vi "Constants.vi"() -> ()   [LabVIEW 2020, in "Ballard MIL-STD-1553 Shared.lvlib"]
doc: "Use this Global VI to access the GUIDs assigned to the page resources of the Custom Device."
uses:
  Ballard MIL-STD-1553 Shared.lvlib
panel:
  in  "Tab Control":enum32{"GUIDs", "Constants", "Properties"}(tab)=enum."Constants"
  in  "RTM Wrapper":string="5FF42902-C783-4304-B588-1D2F1CA49C45"
  in  "Compiled.Settings":string="Compiled.Settings"
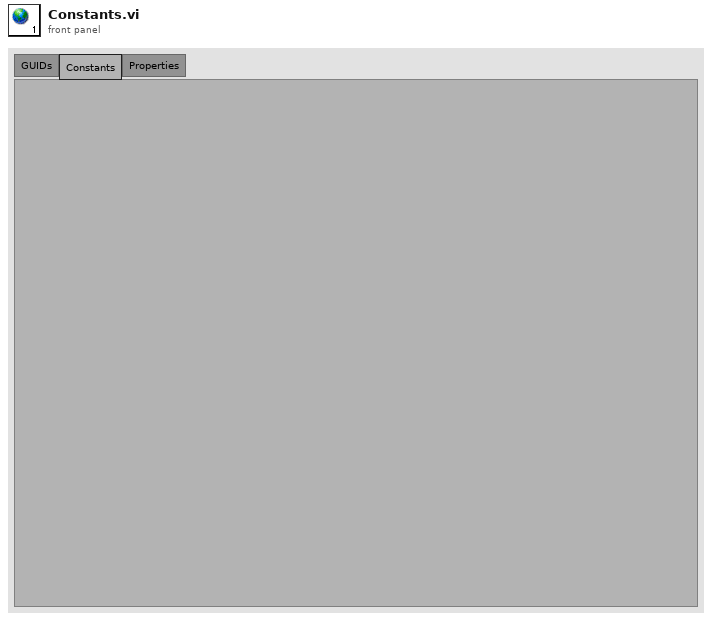
[diagram p1: front panel]
diagram:
